vi "SetChannelsRequest.vi"(8 "error in (no error)":errorcluster, 10 "Channels":T1, 11 "ModuleID":i32) -> (0 "error out":errorcluster)   [LabVIEW 2014, in "FgenPlugins.lvlib" / "FgenPluginsBase.lvclass"]
uses:
  FgenPluginsBase.lvclass
  TypeDefs/Channels.ctl
  TypeDefs/Channel.ctl
  FgenModule/Protected/clEventType.ctl
  <vilib>/Utility/error.llb/Error Cluster From Error Code.vi
  <vilib>/ErrorRing/Error Ring.xnode
  FgenModule/FgenModule.lvlib
  FgenPlugins.lvlib
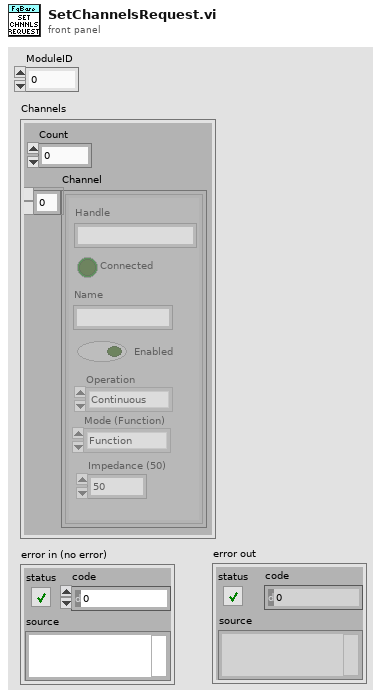
[diagram p1: front panel]
types:
  T1 = typedef "FgenPlugins.lvlib/Channels.ctl" = cluster{"Count":u16, "Channel":T2[]}
  T2 = typedef "FgenPlugins.lvlib/Channel.ctl" = cluster{"Name":string, "Enabled":bool, "Operation":enum16{"Continuous", "Burst"}, "Impedance (50)":dbl, "Handle":string, "Connected":bool, "Mode (Function)":enum16{"Function", "Arbitrary", "Sequence"}}
  T3 = typedef "FgenModule.lvlib/clRequestEvents.ctl" = cluster{"StopRequest":refnum<user-event>, "PathToINI":refnum<user-event>, " LoadPlugin":refnum<user-event>, "ShowPanel":refnum<user-event>, "Initialize":refnum<user-event>, "GetChannels":refnum<user-event>, "SetChannels":refnum<user-event>, "Abort":refnum<user-event>, "Initiate":refnum<user-event>, "ConfigDlg":refnum<user-event>, "GetFunction":refnum<user-event>, "SetFunction":refnum<user-event>, "ConfigFunction":refnum<user-event>, "GetWfrm":refnum<user-event>, "SetWfrm":refnum<user-event>, "GetTriggers":refnum<user-event>, "SetTriggers":refnum<user-event>, "ConfigTriggers":refnum<user-event>}
  T4 = typedef "FgenModule.lvlib/clEventType.ctl" = cluster{"ModuleID":i32, "Data":variant}
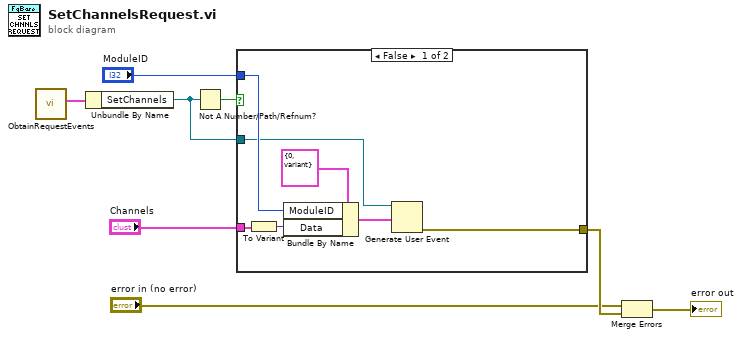
[diagram p0: block diagram]
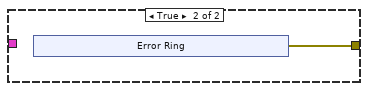
[diagram p2: hidden frame]
diagram:
  n1 = call "ObtainRequestEvents.vi"() -> ("clRequestEvents"=w8:T3)  [unwired: 10 in, 1 out]
  n2 = Unbundle By Name(w8) -> ("SetChannels"=w6:refnum<user-event>)
  n3 = Not A Number/Path/Refnum?(number/path/refnum=w6) -> (NaN/Path/Refnum?=w7:bool)
  n4 = case shown="False" w7 {
    tunnel: w6 -> [w12 _]
    tunnel: "ModuleID" -> [w14 _]
    tunnel: [w11 w16] -> w3
    tunnel: "Channels" -> [w9 _]
    frame False {
      n5 = To Variant(anything=w9) -> (Variant=w10:variant)
      n6 = Bundle By Name(cluster=T4 {"ModuleID"=0, "Data"=variant} ("clEventType"), "ModuleID"=w14, "Data"=w10) -> (w13:T4)
      n7 = Generate User Event(user event=w12, event data cluster=w13) -> (error out=w11:errorcluster)  [unwired: 2 in, 1 out]
    }
    frame True {
      n8 = xnode "Error Ring"() -> ("error out"=w16:errorcluster)
    }
  }
  n9 = Merge Errors("error in (no error)", w3) -> (→"error out":errorcluster)
